vi "calc_phase_map_no_noise.vi"(5 "image name":string="fringe") -> (0 "raw phase map array":u8[][](array[numeric]), 2 "phase map":T1(plugin-control))   [LabVIEW 2011]
uses:
  global_vars.vi
panel:
  in  "y":dbl
  in  "Boolean":bool
  in  "index (row)":i32(slide) scale=0.0..1000.0
  out "Waveform Graph":dbl[][](graph)
  out "i1-i3":dbl[][](graph)
  out "i4-i2":dbl[][](graph)
  in  "u8_pxar_dist":u8[][][](array[numeric])=array4x500x1000[2000000 elements]
  in  "add":dbl
  in  "multi":dbl
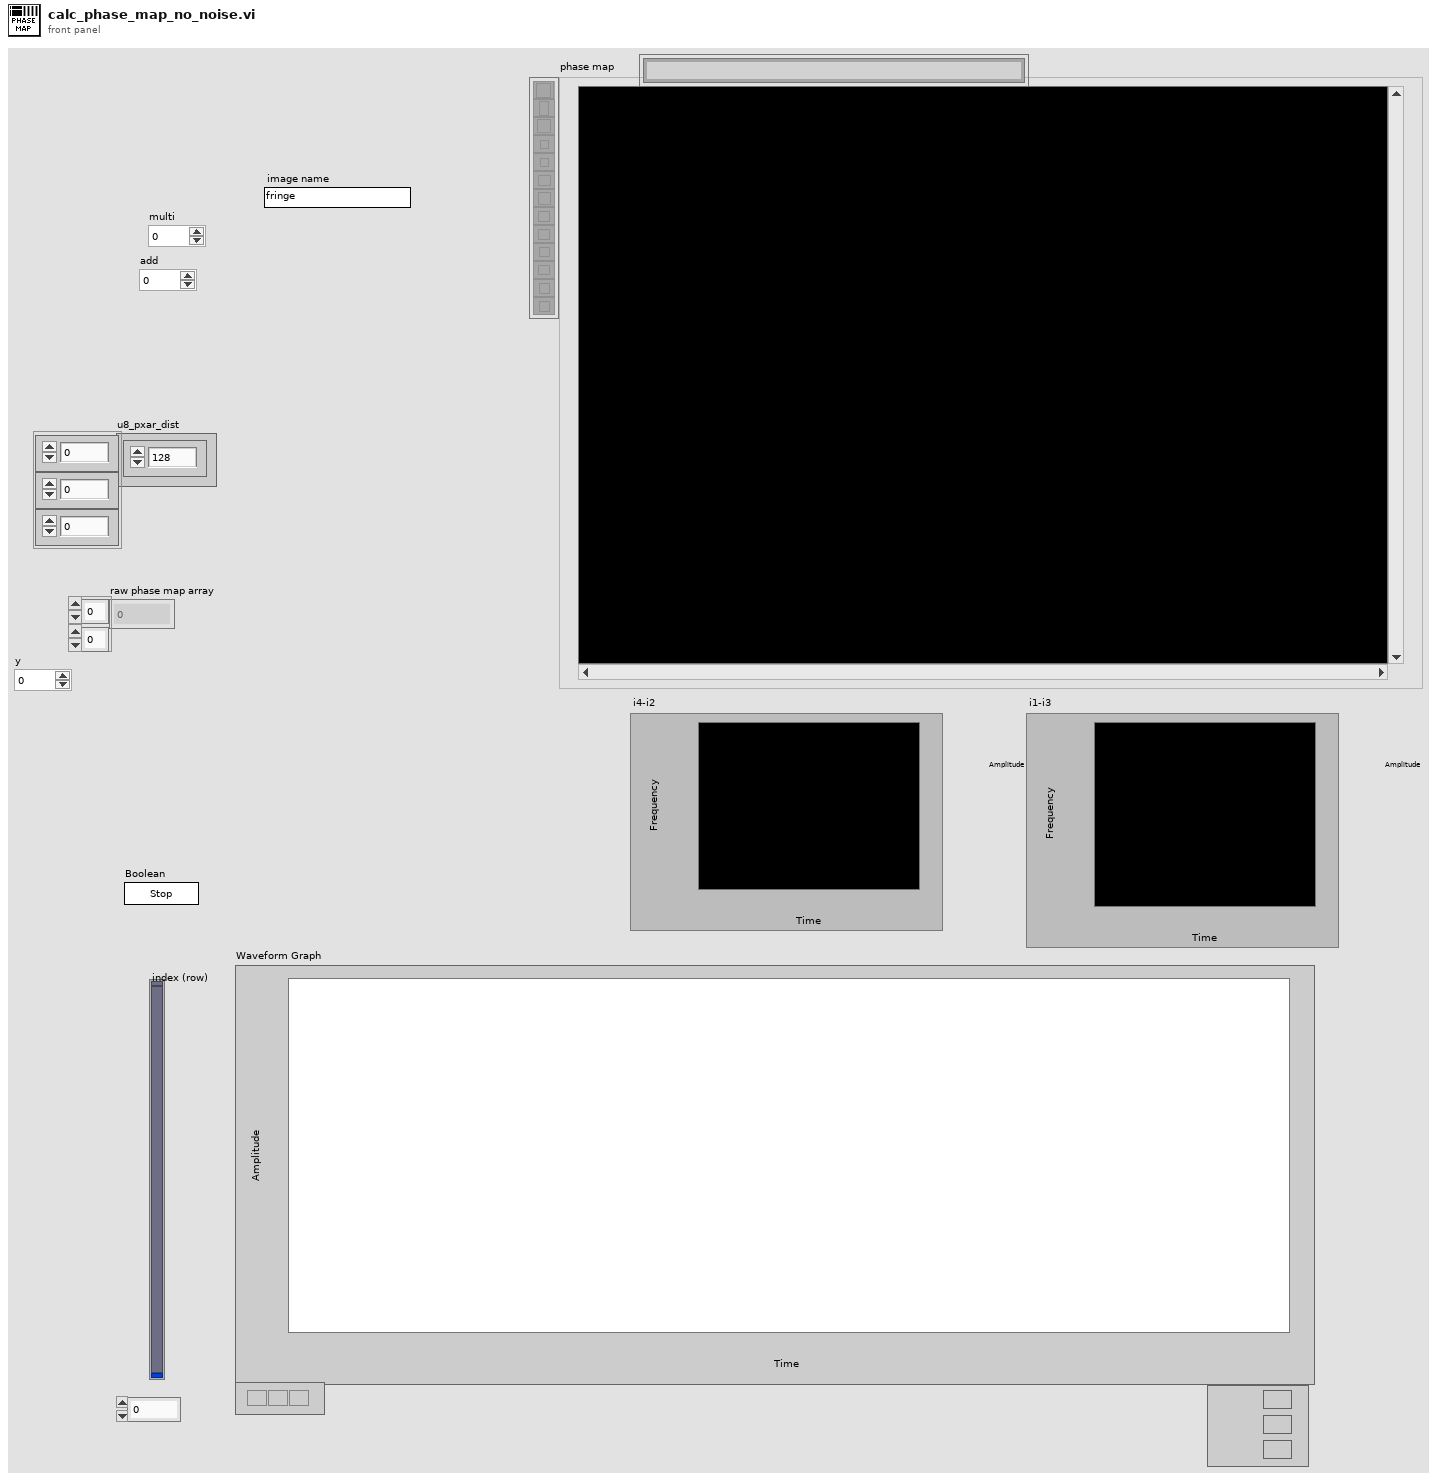
[diagram p1: front panel]
types:
  T1 = typedef "IMAQ Image.ctl" = refnum<image>
  T2 = typedef "Image Type" = u32
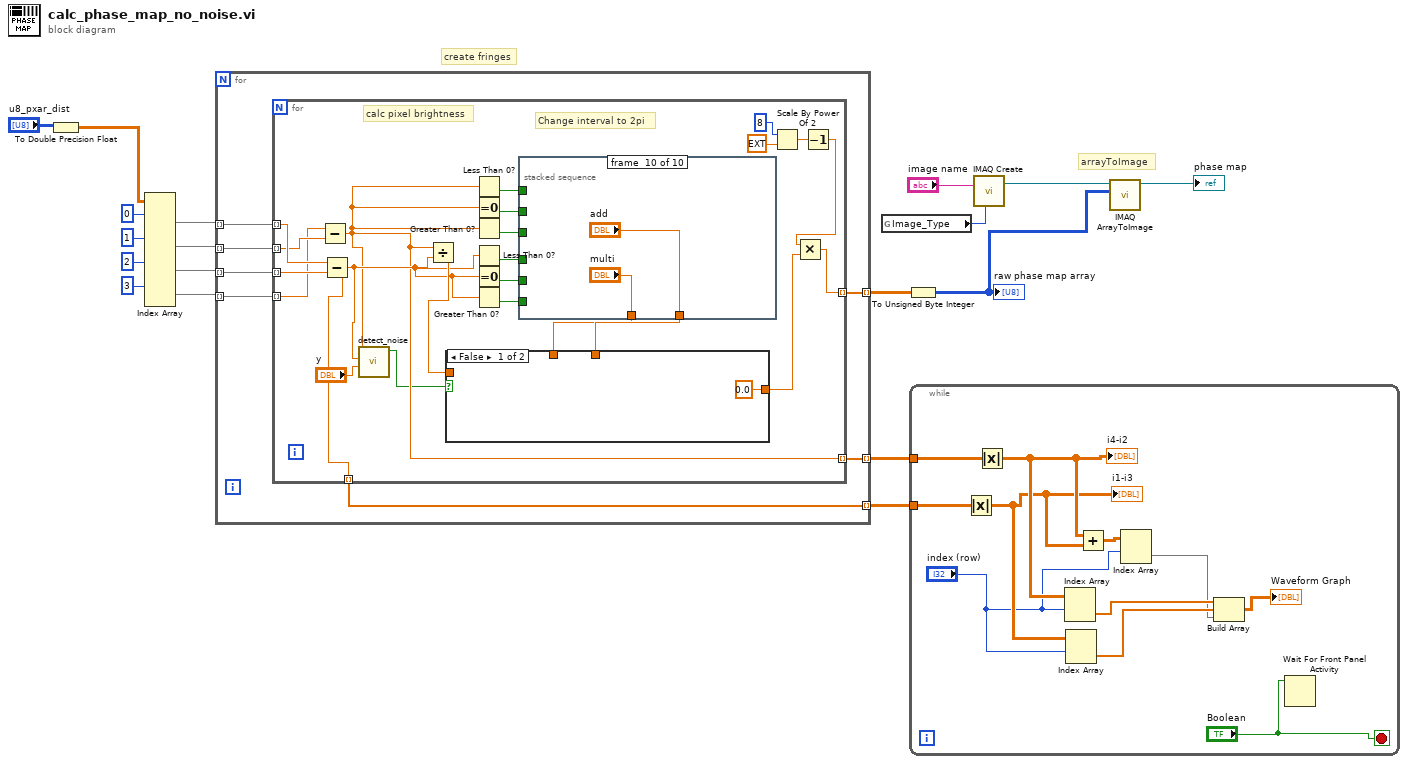
[diagram p0: block diagram]
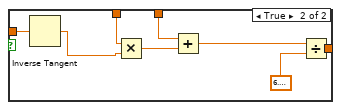
[diagram p2: hidden frame]
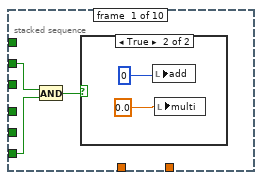
[diagram p3: hidden frame]
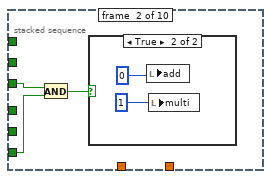
[diagram p5: hidden frame]
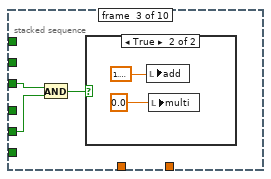
[diagram p7: hidden frame]
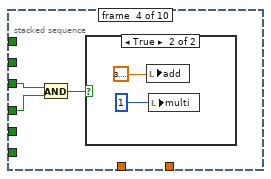
[diagram p9: hidden frame]
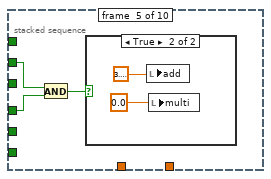
[diagram p11: hidden frame]
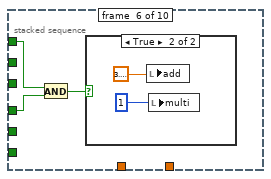
[diagram p13: hidden frame]
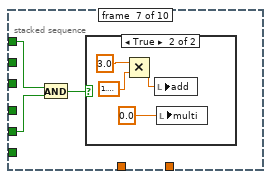
[diagram p15: hidden frame]
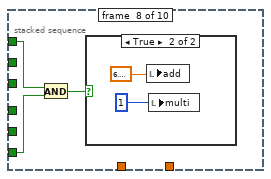
[diagram p17: hidden frame]
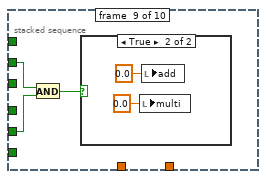
[diagram p19: hidden frame]
diagram:
  # "arrayToImage"
  # "create fringes"
  n1 = To Double Precision Float(number="u8_pxar_dist") -> (double precision float=w3:dbl[][][])
  n2 = Index Array(array=w3, index (dim 0) #1=0 ("index (page)"), index (dim 0) #2=1 ("index (page)"), index (dim 0) #3=2 ("index (page)"), index (dim 0) #4=3 ("index (page)")) -> (element #1=w14:dbl[][], element #2=w13:dbl[][], element #3=w12:dbl[][], element #4=w11:dbl[][])  [unwired: 8 in]
  n3 = for {
    tunnel: w14 -> [w25] mode=indexing
    tunnel: w13 -> [w24] mode=indexing
    tunnel: w12 -> [w23] mode=indexing
    tunnel: w11 -> [w22] mode=indexing
    tunnel: [w21] -> w10 mode=indexing
    tunnel: [w20] -> w2 mode=indexing
    tunnel: [w19] -> w1 mode=indexing
    n4 = for {
      tunnel: w25 -> [w36] mode=indexing
      tunnel: w24 -> [w35] mode=indexing
      tunnel: w23 -> [w32] mode=indexing
      tunnel: w22 -> [w31] mode=indexing
      tunnel: [w44] -> w21 mode=indexing
      tunnel: [w28] -> w20 mode=indexing
      tunnel: [w29] -> w19 mode=indexing
      # "Change interval to 2pi"
      # "calc pixel brightness"
      n5 = Subtract(x=w31, y=w35) -> (x-y=w28:dbl)
      n6 = Subtract(x=w36, y=w32) -> (x-y=w29:dbl)
      n7 = call "detect_noise.vi"("threshold"="y", "i1-i3"=w29, "i4-i2"=w28) -> ("noise/background"=w26:bool)  [unwired: 8 in]
      n8 = Divide(x=w28, y=w29) -> (x/y=w30:dbl)
      n9 = Less Than 0?(x=w28) -> (x < 0?=w42:bool)
      n10 = Equal To 0?(x=w28) -> (x = 0?=w41:bool)
      n11 = Greater Than 0?(x=w28) -> (x > 0?=w40:bool)
      n12 = Less Than 0?(x=w29) -> (x < 0?=w37:bool)
      n13 = Equal To 0?(x=w29) -> (x = 0?=w38:bool)
      n14 = Greater Than 0?(x=w29) -> (x > 0?=w39:bool)
      n15 = stacked-sequence {
        tunnel: w42 -> [_ _ _ _ _ w84 w89 w95 _ _]
        tunnel: w41 -> [w59 _ _ _ w79 _ _ _ w100 _]
        tunnel: w40 -> [_ w64 w68 w74 _ _ _ _ _ _]
        tunnel: w39 -> [w58 w63 _ _ _ _ _ w96 _ _]
        tunnel: w38 -> [_ _ w69 _ _ _ w88 _ w101 _]
        tunnel: w37 -> [_ _ _ w73 w78 w83 _ _ _ _]
        tunnel: [_ _ _ _ _ _ _ _ _ "add"] -> w34
        tunnel: [_ _ _ _ _ _ _ _ _ "multi"] -> w33
        frame #0 {
          n16 = And(x=w59, y=w58) -> (x .and. y?=w60:bool)
          n17 = case shown="True" w60 {
            frame False {
            }
            frame True {
              n18 = local write "add"(0) -> ()
              n19 = local write "multi"(0.0) -> ()
            }
          }
        }
        frame #1 {
          n20 = And(x=w64, y=w63) -> (x .and. y?=w65:bool)
          n21 = case shown="True" w65 {
            frame False {
            }
            frame True {
              n22 = local write "add"(0) -> ()
              n23 = local write "multi"(1) -> ()
            }
          }
        }
        frame #2 {
          n24 = And(x=w68, y=w69) -> (x .and. y?=w70:bool)
          n25 = case shown="True" w70 {
            frame False {
            }
            frame True {
              n26 = local write "add"(1.5707963267948966) -> ()
              n27 = local write "multi"(0.0) -> ()
            }
          }
        }
        frame #3 {
          n28 = And(x=w74, y=w73) -> (x .and. y?=w75:bool)
          n29 = case shown="True" w75 {
            frame False {
            }
            frame True {
              n30 = local write "add"(3.141592653589793) -> ()
              n31 = local write "multi"(1) -> ()
            }
          }
        }
        frame #4 {
          n32 = And(x=w79, y=w78) -> (x .and. y?=w80:bool)
          n33 = case shown="True" w80 {
            frame False {
            }
            frame True {
              n34 = local write "add"(3.141592653589793) -> ()
              n35 = local write "multi"(0.0) -> ()
            }
          }
        }
        frame #5 {
          n36 = And(x=w84, y=w83) -> (x .and. y?=w85:bool)
          n37 = case shown="True" w85 {
            frame False {
            }
            frame True {
              n38 = local write "add"(3.141592653589793) -> ()
              n39 = local write "multi"(1) -> ()
            }
          }
        }
        frame #6 {
          n40 = And(x=w89, y=w88) -> (x .and. y?=w90:bool)
          n41 = case shown="True" w90 {
            frame False {
            }
            frame True {
              n42 = Multiply(x=3.0, y=1.5707963267948966) -> (x*y=w93:dbl)
              n43 = local write "add"(w93) -> ()
              n44 = local write "multi"(0.0) -> ()
            }
          }
        }
        frame #7 {
          n45 = And(x=w95, y=w96) -> (x .and. y?=w97:bool)
          n46 = case shown="True" w97 {
            frame False {
            }
            frame True {
              n47 = local write "add"(6.283185307179586) -> ()
              n48 = local write "multi"(1) -> ()
            }
          }
        }
        frame #8 {
          n49 = And(x=w100, y=w101) -> (x .and. y?=w102:bool)
          n50 = case shown="True" w102 {
            frame False {
            }
            frame True {
              n51 = local write "multi"(0.0 ("multi")) -> ()
              n52 = local write "add"(0.0 ("add")) -> ()
            }
          }
        }
        frame #9 {
        }
      }
      n53 = case shown="False" w26 {
        tunnel: [0.0 w57] -> w45
        tunnel: w34 -> [_ w54]
        tunnel: w33 -> [_ w52]
        tunnel: w30 -> [_ w50]
        frame False {
        }
        frame True {
          n54 = Inverse Tangent(1:w50) -> (0:w51:dbl)
          n55 = Multiply(x=w52, y=w51) -> (x*y=w53:dbl)
          n56 = Add(x=w54, y=w53) -> (x+y=w55:dbl)
          n57 = Divide(x=w55, y=6.283185307179586) -> (x/y=w57:dbl)
        }
      }
      n58 = Scale By Power Of 2(n=8, x=ext 1.0) -> (x*2^n=w47:ext)
      n59 = Decrement(x=w47) -> (x-1=w46:ext)
      n60 = Multiply(x=w46, y=w45) -> (x*y=w44:ext)
    }
  }
  n61 = global read "global_vars.vi" "Image_Type"() -> (w6:T2)
  n62 = To Unsigned Byte Integer(number=w10) -> (unsigned 8bit integer=w5:u8[][])
  "raw phase map array" <- w5
  n63 = while {
    tunnel: w2 -> [w112]
    tunnel: w1 -> [w117]
    stop <- "Boolean" stop-if-true
    n64 = Absolute Value(x=w117) -> (abs(x)=w110:dbl[][])
    "i1-i3" <- w110
    n65 = Absolute Value(x=w112) -> (abs(x)=w111:dbl[][])
    "i4-i2" <- w111
    n66 = Index Array(array=w111, index (row)="index (row)") -> (element=w116:dbl[])  [unwired: 1 in]
    n67 = Index Array(array=w110, index (row)="index (row)") -> (element=w115:dbl[])  [unwired: 1 in]
    n68 = Add(x=w111, y=w110) -> (x+y=w109:dbl[][])
    n69 = Index Array(array=w109, index (row)="index (row)") -> (element=w107:dbl[])  [unwired: 1 in]
    n70 = Build Array(w116, w115, w107) -> (→"Waveform Graph":dbl[][])
    n71 = Wait For Front Panel Activity(3:"Boolean") -> ()  [unwired: 2 in, 1 out]
  }
  n72 = call "IMAQ Create"("Image Name"="image name", "Image Type"=w6) -> ("New Image"=w7:T1)  [unwired: 2 in, 2 out]
  n73 = call "IMAQ ArrayToImage"("Image Pixels (U8)"=w5, "Image"=w7) -> ("Image Out"=→"phase map":T1)  [unwired: 8 in, 1 out]
